vi "Calculate Velocities.vi"(1 "Path Direction Info":T2, 2 "Angular Data (Relative)":dbl[](array[numeric])=[0.0, 0.0, 0.0, 0.0, 0.0, 0.0, 0.0, 0.0, 0.0, 0.0, 0.0, 0.0, 0.0, 0.0, 0.0, 0.0, 0.0, 0.0, 0.0, 0.0, 0.0, 0.0, 0.0, 0.0, 0.0, 0.0, 0.0, 0.0, 0.0, -0.16103332399232784, -0.2660653812379792, -0.3711094905327599, -0.47616115663132064, -0.5811932138769862, -0.6862252711226517, -0.7912814324665192, -0.8963210465159932, -1.0013531037616588, -1.1063896562526168, -1.2114488791550002, -1.3164809364006516, -1.4215129936463171, -1.5265615981863903, -1.6316087690396728, -1.73664082628531, -1.8416728835309897, -1.946733540120178, -2.051768658924317, -2.1568007161699967, -2.2618417639062613, -2.366896491563331, -2.4719285488089966, -2.576960606054641, -2.682013705840042, -2.7870563814480036, -2.892088438693655, -2.9971219296261324, -2.924737139700433, -2.923227086540436, -2.8181950292947846, -2.7131494863132133, -2.6080992539014503, -2.503067196655749, -2.398035139410112, -2.2929775443794327, -2.187939364016785, -2.082907306771105, -1.9778693205933422, -1.8728115313777636, -1.767779474132098, -1.6627474168864325, -1.5576973786595687, -1.4526516414931052, -1.3476195842474397, -1.242587527001774, -1.137525436725781, -1.0324917516084327, -0.9274596943627813, -0.8224172129396976, -0.7173639189694256, -0.6123318617237601, -0.507299804478123, -0.4022452710059241, -0.2972040290847531, -0.19217197183908752, -0.08713704721984072, -0.0056450421224099046, 0.0, 0.0, 0.0, -0.21964882672565256, -0.36338830970408753, -0.5071186597231498, -0.6508388775735292, -0.7945884927206468, -0.9382995776116538, -1.0820481935494604, -1.2257694106091481, -1.369498761418905, -1.5132392436066482, -1.656950328497647, -1.8007080773948374, -1.9444201614951524, -2.0881586452642775, -2.2318899944926507, -2.3756092131337176, -2.519359827490142, -2.6630709123811585, -2.806818529109659, -2.950540745378639, -3.094269096979101, -3.238010578376148, -3.3817216632671574, -3.409046053670437, -3.42889375340539, -3.285156268845597, -3.1414239204079024, -2.997705700976134, -2.8539540874104077, -2.7102430025194053, -2.5664963850002067, -2.4227731695219177, -2.279045817130765, -2.1353033365244016, -1.9915922516333922, -1.8478365011548306, -1.7041224186359045, -1.5603859332854029, -1.4166525856383885, -1.272935365415961, -1.129182752640915, -0.9854716677498914, -0.8417260494400125, -0.6980018347524037, -0.5542754815705848, -0.4105320017549161, -0.2668209168638782, -0.12306616559465056, -0.009079861230148367, 0.0, 0.0, 0.0, -0.20470865860326626, -0.33856329496950366, -0.47241793133574106, -0.6062725677019642, -0.7401349766972771, -0.8740022344657774, -1.0078568708320148, -1.1417115071982522, -1.2755661435644754, -1.4094207799306986, -1.5432909615551296, -1.677150446694526, -1.8110050830607634, -1.9448597194269865, -2.078714355793224, -2.212571916015378, -2.3464440225570513, -2.4802986589232745, -2.614153295289512, -2.748007931655735, -2.8818625680219725, -3.0157279008732303, -3.1495922347857714, -3.2834468711520373, -3.4173015075182605, -3.404811406362427, -3.3999504519296693, -3.26607734644935, -3.1322207851658277, -2.9983661487996187, -2.8645115124334097, -2.7306568760671723, -2.5967963919890735, -2.4629272093033023, -2.3290725729370934, -2.195217936570913, -2.061363300204647, -1.9275086638384096, -1.793640407131221, -1.6597789970745964, -1.525924360708359, -1.3920697243420932, -1.2582150879759126, -1.1243594526710012, -0.9904854212120711, -0.8566307848458337, -0.7227761484796247, -0.5889215121133589, -0.4550668757471499, -0.3212034678131772, -0.1873372089833083, -0.05411439755982883, 0.0, 0.0, 0.0, 0.0, 0.0, 0.0, 0.0, 0.0, 0.0, -0.23219985680768218, -0.384231932551927, -0.5362507909605654, -0.6882652353272647, -0.8403017251134486, -0.992302952144513, -1.1443482452244496, -1.2963538862973962, -1.4483815479997872, -1.6004048204503079, -1.7524148507750965, -1.9044557546032195, -2.0564569816342555, -2.2084978606722814, -2.360507915787167, -2.512531163447619, -2.6645588499400503, -2.8165644662229568, -2.968609784092962, -3.1206110111240264, -3.272647476120113, -3.424661945276938, -3.576680778895451, -3.52404056310354, -3.4776533617836094, -3.3256036794518593, -3.1736024276306836, -3.021570376676536, -2.8695514934778146, -2.717537073901198, -2.565500559324917, -2.4134993322938385, -2.2614540640040417, -2.109448398140941, -1.9574207612286756, -1.805397463988072, -1.653387458453338, -1.5013465298351605, -1.3493453028040818, -1.1973044485561957, -1.0452943686511986, -0.8932711457808438, -0.741243434498287, -0.5892378430055061, -0.437192500345418, -0.28519127331433936, -0.13315483310833542, -0.010697299143600958, 0.0, 0.0, 0.0], 3 "Velocities":dbl[](array[numeric])=[0.06, 0.18, 0.36, 0.6, 0.8999999999999999, 1.2, 1.5, 1.8, 2.1, 2.4, 2.6999999999999997, 2.9999999999999996, 3.2999999999999994, 3.599999999999999, 3.899999999999999, 4.199999999999999, 4.499999999999999, 4.799999999999999, 5.099999999999999, 5.399999999999999, 5.699999999999998, 5.999999999999998, 6.299999999999998, 6.599999999999998, 6.899999999999998, 7.1999999999999975, 7.439999999999998, 7.619999999999997, 7.619999999999997, 7.619999999999997, 7.619999999999997, 7.619999999999997, 7.619999999999997, 7.619999999999997, 7.619999999999997, 7.619999999999997, 7.619999999999997, 7.619999999999997, 7.619999999999997, 7.619999999999997, 7.619999999999997, 7.619999999999997, 7.619999999999997, 7.619999999999997, 7.619999999999997, 7.619999999999997, 7.619999999999997, 7.619999999999997, 7.619999999999997, 7.619999999999997, 7.619999999999997, 7.619999999999997, 7.619999999999997, 7.619999999999997, 7.619999999999997, 7.619999999999997, 7.619999999999997, 7.619999999999997, 7.619999999999997, 7.619999999999997, 7.619999999999997, 7.619999999999997, 7.619999999999997, 7.619999999999997, 7.619999999999997, 7.619999999999997, 7.619999999999997, 7.619999999999997, 7.619999999999997, 7.619999999999997, 7.619999999999997, 7.619999999999997, 7.619999999999997, 7.619999999999997, 7.619999999999997, 7.619999999999997, 7.619999999999997, 7.619999999999997, 7.619999999999997, 7.619999999999997, 7.619999999999997, 7.619999999999997, 7.619999999999997, 7.619999999999997, 7.619999999999997, 7.619999999999997, 7.619999999999997, 7.619999999999997, 7.619999999999997, 7.619999999999997, 7.619999999999997, 7.619999999999997, 7.619999999999997, 7.619999999999997, 7.619999999999997, 7.619999999999997, 7.619999999999997, 7.619999999999997, 7.619999999999997, 7.619999999999997, 7.619999999999997, 7.619999999999997, 7.619999999999997, 7.619999999999997, 7.619999999999997, 7.619999999999997, 7.619999999999997, 7.619999999999997, 7.619999999999997, 7.619999999999997, 7.619999999999997, 7.619999999999997, 7.619999999999997, 7.619999999999997, 7.619999999999997, 7.619999999999997, 7.619999999999997, 7.619999999999997, 7.619999999999997, 7.619999999999997, 7.619999999999997, 7.619999999999997, 7.619999999999997, 7.619999999999997, 7.619999999999997, 7.619999999999997, 7.619999999999997, 7.619999999999997, 7.619999999999997, 7.619999999999997, 7.619999999999997, 7.619999999999997, 7.619999999999997, 7.619999999999997, 7.619999999999997, 7.619999999999997, 7.619999999999997, 7.619999999999997, 7.619999999999997, 7.619999999999997, 7.619999999999997, 7.619999999999997, 7.619999999999997, 7.619999999999997, 7.619999999999997, 7.619999999999997, 7.619999999999997, 7.619999999999997, 7.619999999999997, 7.619999999999997, 7.619999999999997, 7.619999999999997, 7.619999999999997, 7.619999999999997, 7.619999999999997, 7.619999999999997, 7.619999999999997, 7.619999999999997, 7.619999999999997, 7.619999999999997, 7.619999999999997, 7.619999999999997, 7.619999999999997, 7.619999999999997, 7.619999999999997, 7.619999999999997, 7.619999999999997, 7.619999999999997, 7.619999999999997, 7.619999999999997, 7.619999999999997, 7.619999999999997, 7.619999999999997, 7.619999999999997, 7.619999999999997, 7.619999999999997, 7.619999999999997, 7.619999999999997, 7.619999999999997, 7.619999999999997, 7.619999999999997, 7.619999999999997, 7.619999999999997, 7.619999999999997, 7.619999999999997, 7.619999999999997, 7.619999999999997, 7.619999999999997, 7.619999999999997, 7.619999999999997, 7.619999999999997, 7.619999999999997, 7.619999999999997, 7.619999999999997, 7.619999999999997, 7.619999999999997, 7.619999999999997, 7.619999999999997, 7.619999999999997, 7.619999999999997, 7.619999999999997, 7.619999999999997, 7.619999999999997, 7.619999999999997, 7.619999999999997, 7.619999999999997, 7.619999999999997, 7.619999999999997, 7.619999999999997, 7.619999999999997, 7.619999999999997, 7.619999999999997, 7.619999999999997, 7.619999999999997, 7.619999999999997, 7.619999999999997, 7.619999999999997, 7.619999999999997, 7.619999999999997, 7.619999999999997, 7.619999999999997, 7.619999999999997, 7.619999999999997, 7.619999999999997, 7.619999999999997, 7.619999999999997, 7.619999999999997, 7.619999999999997, 7.619999999999997, 7.619999999999997, 7.619999999999997, 7.619999999999997, 7.619999999999997, 7.619999999999997, 7.619999999999997, 7.619999999999997, 7.619999999999997, 7.619999999999997, 7.619999999999997, 7.619999999999997, 7.619999999999997, 7.619999999999997, 7.619999999999997, 7.619999999999997, 7.619999999999997, 7.619999999999997, 7.619999999999997, 7.619999999999997, 7.619999999999997, 7.619999999999997, 7.619999999999997, 7.319999999999998, 7.019999999999998, 6.719999999999998], 5 "Iteration":i32=255, 6 "IMU Input":dbl=-78.43260738413034, 7 "Start Time":i32=4558415, 8 "PID gains":T1={"proportional gain (Kc)"=0.2, "integral time (Ti, min)"=0.0001, "derivative time (Td, min)"=0.0001} {"derivative time (Td, min)" format="%.3f"; "integral time (Ti, min)" format="%.3f"; "proportional gain (Kc)" format="%.3f"}) -> (13 "Desired Angle (Absolute)":dbl=-359.18362432782453, 14 "Left Velocity":dbl=38375.0, 16 "Right Velocity":dbl=-38375.0, 17 "Finished?":bool=TRUE, 19 "Wait Time":i32=7)   [LabVIEW 2019]
panel:
  in  "Conversion to SparkMax Units":dbl=383.75
  in  "Enable IMU":bool=TRUE
  in  "Angular Component":dbl=80.0
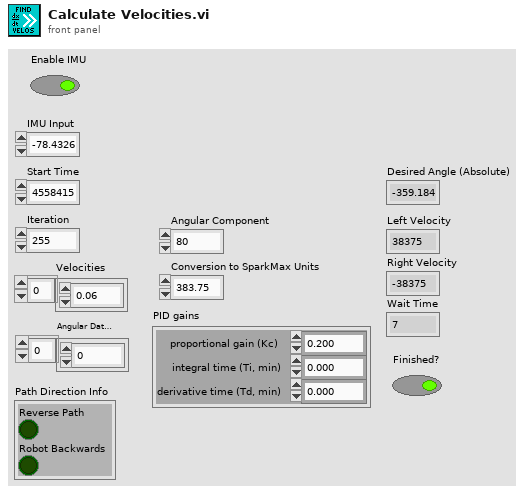
[diagram p1: front panel]
types:
  T1 = cluster{"proportional gain (Kc)":dbl, "integral time (Ti, min)":dbl, "derivative time (Td, min)":dbl}
  T2 = cluster{"Reverse Path":bool, "Robot Backwards":bool}
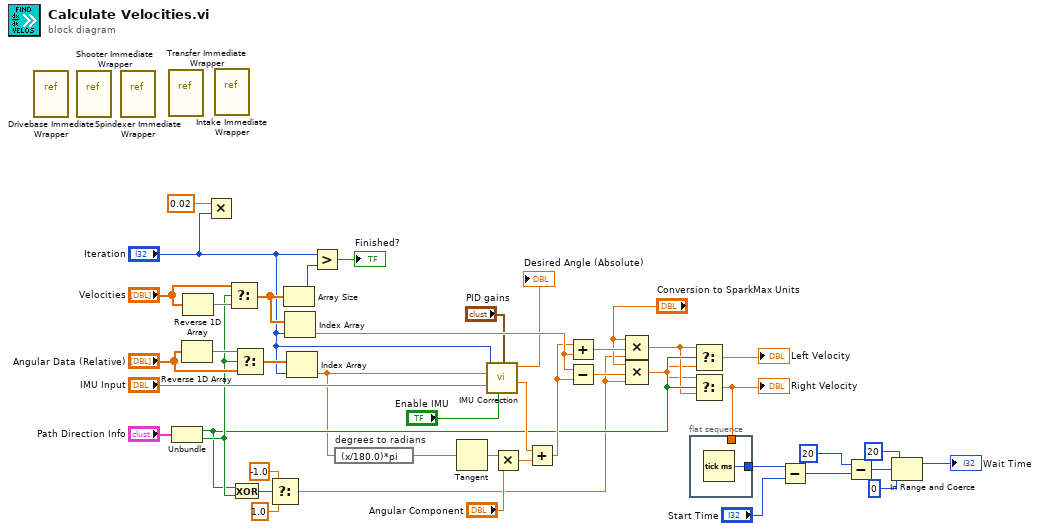
[diagram p0: block diagram]
diagram:
  n1 = vi-ref "Drivebase Immediate Wrapper.vi"() -> ()  [unwired: 1 out]
  n2 = vi-ref "Shooter Immediate Wrapper.vi"() -> ()  [unwired: 1 out]
  n3 = vi-ref "Spindexer Immediate Wrapper.vi"() -> ()  [unwired: 1 out]
  n4 = vi-ref "Transfer Immediate Wrapper.vi"() -> ()  [unwired: 1 out]
  n5 = Unbundle("Path Direction Info") -> ("Reverse Path"=w22:bool, "Robot Backwards"=w25:bool)
  n6 = Reverse 1D Array(array="Angular Data (Relative)") -> (reversed array=w29:dbl[])
  n7 = Reverse 1D Array(array="Velocities") -> (reversed array=w32:dbl[])
  n8 = Multiply(x=0.02, y="Iteration") -> ()  [unwired: 1 out]
  n9 = vi-ref "Intake Immediate Wrapper.vi"() -> ()  [unwired: 1 out]
  n10 = Select(t="Velocities", s=w25, f=w32) -> (s? t:f=w30:dbl[])
  n11 = Exclusive Or(1:w25, 2:w22) -> (0:w26:bool)
  n12 = Select(t=w29, s=w25, f="Angular Data (Relative)") -> (s? t:f=w27:dbl[])
  n13 = Select(t=-1.0, s=w26, f=1.0) -> (s? t:f=w8:dbl)
  n14 = Array Size(array=w30) -> (size(s)=w34:i32)
  n15 = Index Array(array=w30, index="Iteration") -> (element=w42:dbl)
  n16 = Index Array(array=w27, index="Iteration") -> (element=w17:dbl)
  n17 = Greater?(x="Iteration", y=w34) -> (0:→"Finished?":bool)
  n18 = expression code="(x/180.0)*pi" "degrees to radians"(w17) -> (w16:dbl)
  n19 = Tangent(1:w16) -> (0:w15:dbl)
  n20 = call "IMU Correction.vi"("Enable IMU"="Enable IMU", "Current Angle"="IMU Input", "Desired Angle (Relative)"=w17, "Iterations"="Iteration", "PID gains"="PID gains") -> ("IMU Correction"=w36:dbl, "Desired Angle (Absolute)"=→"Desired Angle (Absolute)":dbl)  [unwired: 5 in]
  n21 = Multiply(x=w15, y="Angular Component") -> (x*y=w37:dbl)
  n22 = Add(x=w36, y=w37) -> (x+y=w35:dbl)
  n23 = Add(x=w35, y=w42) -> (x+y=w21:dbl)
  n24 = Subtract(x=w42, y=w35) -> (x-y=w19:dbl)
  n25 = Compound Arithmetic op=MULTIPLY("Conversion to SparkMax Units", w21, w8) -> (w20:dbl)
  n26 = Compound Arithmetic op=MULTIPLY("Conversion to SparkMax Units", w19, w8) -> (w18:dbl)
  n27 = flat-sequence {
    tunnel: [w45] -> w41
    tunnel: w10 -> [_]
    frame #0 {
      n28 = Tick Count (ms)() -> (millisecond timer value=w45:u32)
    }
  }
  n29 = Select(t=w20, s=w22, f=w18) -> (s? t:f=→"Left Velocity":dbl)
  n30 = Select(t=w18, s=w22, f=w20) -> (s? t:f=w10:dbl)
  "Right Velocity" <- w10
  n31 = Subtract(x=w41, y="Start Time") -> (x-y=w13:u32)
  n32 = Subtract(x=u32 20, y=w13) -> (x-y=w7:u32)
  n33 = In Range and Coerce(upper limit=u32 20, x=w7, lower limit=u32 0) -> (coerced(x)=→"Wait Time":u32)  [unwired: 1 out]
